vi "Blowfish Encipher Decipher.vi"(0 "Xl":u32, 1 "Xr":u32, 2 "P 18":u32[](array[numeric]), 3 "S 4X256":u32[][](array[numeric]), 4 "Enc/Dec":enum16{"Encipher", "Decipher"}(ring)) -> (5 "Xl out":u32, 6 "Xr out":u32)   [LabVIEW 2022 SP3, in "Registration.lvclass"]
uses:
  Registration.lvclass
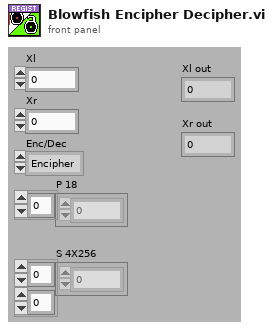
[diagram p1: front panel]
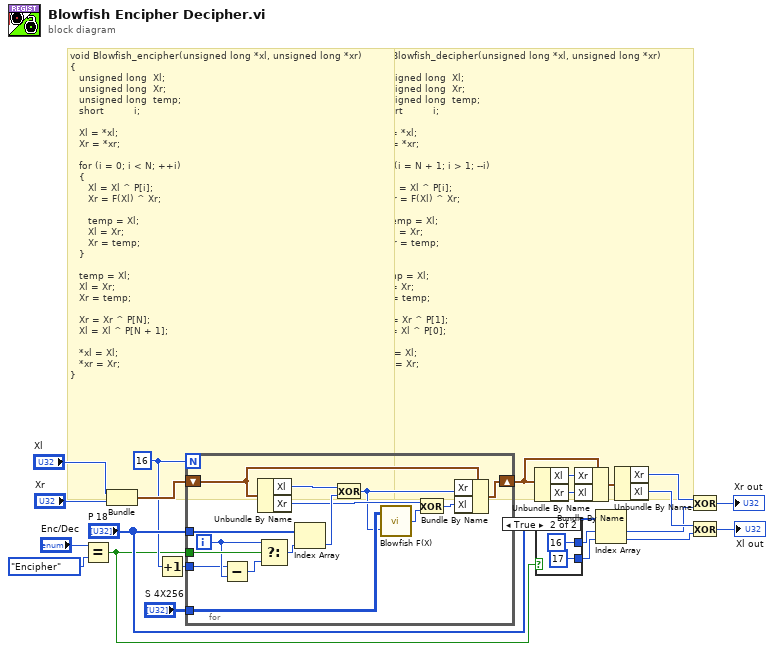
[diagram p0: block diagram]
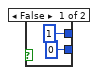
[diagram p2: hidden frame]
diagram:
  w5 = 16
  # "void Blowfish_decipher(unsigned long *xl, unsigned long *xr)\n{\n   unsigned long  Xl;\n   unsigned long  Xr;\n   unsigned long  temp;\n   short          i;\n\n   Xl = *xl;\n   Xr = *xr;\n\n   for (i = N + 1; i > 1; --i)\n   {\n      Xl = Xl ^ P[i];\n      Xr = F(Xl) ^ Xr;\n\n      temp = Xl;\n      Xl = Xr;\n      Xr = temp;\n   }\n\n   temp = Xl;\n   Xl = Xr;\n   Xr = temp;\n\n   Xr = Xr ^ P[1];\n   Xl = Xl ^ P[0];\n\n   *xl = Xl;\n   *xr = Xr;\n}"
  # "void Blowfish_encipher(unsigned long *xl, unsigned long *xr)\n{\n   unsigned long  Xl;\n   unsigned long  Xr;\n   unsigned long  temp;\n   short          i;\n\n   Xl = *xl;\n   Xr = *xr;\n\n   for (i = 0; i < N; ++i)\n   {\n      Xl = Xl ^ P[i];\n      Xr = F(Xl) ^ Xr;\n\n      temp = Xl;\n      Xl = Xr;\n      Xr = temp;\n   }\n\n   temp = Xl;\n   Xl = Xr;\n   Xr = temp;\n\n   Xr = Xr ^ P[N];\n   Xl = Xl ^ P[N + 1];\n\n   *xl = Xl;\n   *xr = Xr;\n}"
  n1 = Equal?(x="Enc/Dec", y=enum16{"Encipher", "Decipher"}."Encipher") -> (x = y?=w2:bool)
  n2 = Bundle("Xl"="Xl", "Xr"="Xr") -> (w10:cluster{"Xl":u32, "Xr":u32})  [unwired: 1 in]
  n3 = Increment(x=w5) -> (x+1=w6:i32)
  n4 = for {
    N: w5 -> [_]
    shift-right: [w30] -> w13
    shift-left: w10 -> [w31]
    tunnel: "P 18" -> [w37]
    tunnel: "S 4X256" -> [w35]
    tunnel: w2 -> [w27]
    tunnel: w6 -> [w23]
    i -> [w24]
    n5 = Subtract(x=w23, y=w24) -> (x-y=w25:i32)
    n6 = Unbundle By Name(w31) -> ("Xl"=w33:u32, "Xr"=w32:u32)
    n7 = Select(t=w24, s=w27, f=w25) -> (s? t:f=w26:i32)
    n8 = Index Array(array=w37, index=w26) -> (element=w36:u32)
    n9 = Exclusive Or(1:w36, 2:w33) -> (0:w29:u32)
    n10 = call "Blowfish F(X).vi"("X"=w29, "S 4X256"=w35) -> ("F(X)"=w34:u32)
    n11 = Exclusive Or(1:w34, 2:w32) -> (0:w28:u32)
    n12 = Bundle By Name(cluster=w31, "Xr"=w29, "Xl"=w28) -> (w30:cluster{"Xl":u32, "Xr":u32})
  }
  n13 = Unbundle By Name(w13) -> ("Xl"=w14:u32, "Xr"=w15:u32)
  n14 = case shown="True" w2 {
    tunnel: [0 ("f") 17 ("f")] -> w4
    tunnel: [1 ("f") 16 ("f")] -> w3
    frame False {
    }
    frame True {
    }
  }
  n15 = Bundle By Name(cluster=w13, "Xr"=w14, "Xl"=w15) -> (w16:cluster{"Xl":u32, "Xr":u32})
  n16 = Index Array(array="P 18", index #1=w3, index #2=w4) -> (element #1=w18:u32, element #2=w1:u32)
  n17 = Unbundle By Name(w16) -> ("Xr"=w17:u32, "Xl"=w20:u32)
  n18 = Exclusive Or(1:w18, 2:w17) -> (0:→"Xr out":u32)
  n19 = Exclusive Or(1:w1, 2:w20) -> (0:→"Xl out":u32)
